vi "Tosca-Layout AI.vi"(0 "Digital":refnum<vi>, 1 "DigitalPane":refnum<vi>, 2 "AnalogPane":refnum<vi>, 5 "Analog":refnum<vi>, 9 "Status":refnum<vi>, 11 "More":refnum<vi>) -> ()   [LabVIEW 2020]
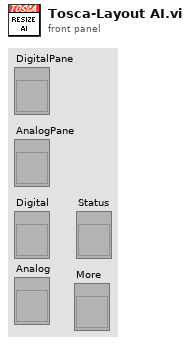
[diagram p1: front panel]
types:
  T1 = typedef "LVBoundsTypeDef.ctl" = cluster{"Width":u32, "Height":u32}
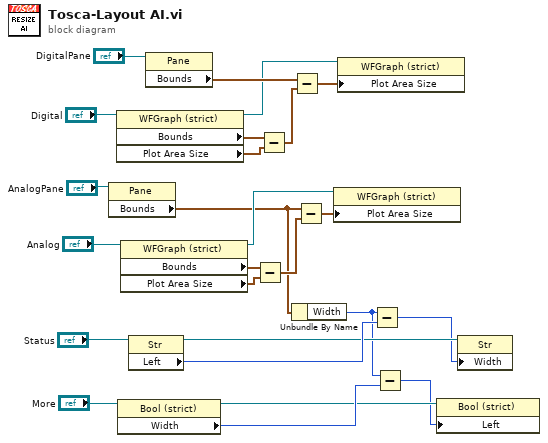
[diagram p0: block diagram]
diagram:
  n1 = property class="Pane"(reference="AnalogPane") -> ("Bounds"=w9:T1)  [unwired: 1 in, 2 out]
  n2 = property class="WFGraph (strict)"(reference="Digital") -> (reference out=w23:refnum<vi>, "Bounds"=w21:T1, "Plot Area Size"=w20:T1)  [unwired: 1 in, 1 out]
  n3 = property on="Property Node" class="Bool (strict)"(reference="More") -> (reference out=w2:refnum<vi>, "Width"=w3:u32)  [unwired: 1 in, 1 out]
  n4 = property class="WFGraph (strict)"(reference="Analog") -> (reference out=w17:refnum<vi>, "Bounds"=w15:T1, "Plot Area Size"=w14:T1)  [unwired: 1 in, 1 out]
  n5 = property class="Str"(reference="Status") -> (reference out=w7:refnum<vi>, "Left"=w8:i32)  [unwired: 1 in, 1 out]
  n6 = property class="Pane"(reference="DigitalPane") -> ("Bounds"=w25:T1)  [unwired: 1 in, 2 out]
  n7 = Subtract(x=w15, y=w14) -> (x-y=w13:T1)
  n8 = Subtract(x=w21, y=w20) -> (x-y=w19:T1)
  n9 = Subtract(x=w25, y=w19) -> (x-y=w22:T1)
  n10 = Unbundle By Name(w9) -> ("Width"=w4:u32)
  n11 = Subtract(x=w9, y=w13) -> (x-y=w16:T1)
  n12 = property class="WFGraph (strict)"(reference=w17, "Plot Area Size"=w16) -> ()  [unwired: 1 in, 2 out]
  n13 = property class="WFGraph (strict)"(reference=w23, "Plot Area Size"=w22) -> ()  [unwired: 1 in, 2 out]
  n14 = Subtract(x=w4, y=w8) -> (x-y=w6:u32)
  n15 = Subtract(x=w4, y=w3) -> (x-y=w1:u32)
  n16 = property class="Bool (strict)"(reference=w2, "Left"=w1) -> ()  [unwired: 1 in, 2 out]
  n17 = property class="Str"(reference=w7, "Width"=w6) -> ()  [unwired: 1 in, 2 out]
